vi "stabilizePress_01.vi"() -> ()   [LabVIEW 2011]
uses:
  <vilib>/Platform/TimedLoop/XDataNode/timing_clust.ctl
  <vilib>/Platform/TimedLoop/XDataNode/nitl_modes.ctl
  <vilib>/Platform/TimedLoop/XDataNode/wakeup.ctl
  <vilib>/Platform/TimedLoop/XDataNode/XDataNode.xnode
  <vilib>/Platform/TimedLoop/XDataNode/XDNodeRunTimeDep.lvlib
  <vilib>/Analysis/NI_AALPro.lvlib
panel:
  in  "dtRamp (s)":i64=2
  in  "local when done":bool=TRUE
  out "Best Exponential Fit":dbl[](array[numeric])=[20.391769446914367, 19.671893548435698, 19.339647975340863, 19.18630609922805, 19.115533956951577, 19.082870367269678, 19.067795084021366, 19.060832753073868, 19.057626153023538, 19.056144077997605, 19.055460053338074, 19.055144354249524, 19.05499864910115, 19.054931401551084, 19.054900364672562, 19.05488604016814, 19.054879428954745, 19.05487637564856, 19.054874969405184, 19.054874319446302, 19.05487401946965, 19.054873881020907]
  out "XY Graph":cluster{"Value":dbl[], "Value":dbl[]}[](graph)=[{"Value"=[1.0, 2.0, 3.0, 4.0, 5.0, 6.0, 7.0, 8.001, 9.0, 10.0, 11.0, 12.0, 13.0, 14.0, 15.0, 16.0, 17.0, 18.001, 19.0, 20.0, 21.0, 22.0], "Value"=[20.39, 19.689999999999998, 19.299999999999997, 19.189999999999998, 19.130000000000003, 19.110000000000003, 19.09, 19.08, 19.07, 19.05, 19.04, 19.04, 19.05, 19.05, 19.05, 19.04, 19.05, 19.060000000000002, 19.060000000000002, 19.05, 19.05, 19.05]}, {"Value"=[1.0, 2.0, 3.0, 4.0, 5.0, 6.0, 7.0, 8.001, 9.0, 10.0, 11.0, 12.0, 13.0, 14.0, 15.0, 16.0, 17.0, 18.001, 19.0, 20.0, 21.0, 22.0], "Value"=[20.391769446914367, 19.671893548435698, 19.339647975340863, 19.18630609922805, 19.115533956951577, 19.082870367269678, 19.067795084021366, 19.060832753073868, 19.057626153023538, 19.056144077997605, 19.055460053338074, 19.055144354249524, 19.05499864910115, 19.054931401551084, 19.054900364672562, 19.05488604016814, 19.054879428954745, 19.05487637564856, 19.054874969405184, 19.054874319446302, 19.05487401946965, 19.054873881020907]}]
  out "Pfinal (torr)":dbl=19.054873762353765
  out "tune done":bool=TRUE
  in  "max dP step (torr)":dbl=0.1
  out "dP(torr)":dbl
  out "amplitude":dbl=2.8966495268264136
  out "damping":dbl=-0.7732044604437537
  out "tune Setpoint(torr)":dbl=20.0
  in  "t array":dbl[](array[numeric])=[1.0, 2.0, 3.0, 4.0, 5.0, 6.0, 7.0, 8.001, 9.0, 10.0, 11.0, 12.0, 13.0, 14.0, 15.0, 16.0, 17.0, 18.001, 19.0, 20.0, 21.0, 22.0]
  out "P array":dbl[](array[numeric])=[20.39, 19.689999999999998, 19.299999999999997, 19.189999999999998, 19.130000000000003, 19.110000000000003, 19.09, 19.08, 19.07, 19.05, 19.04, 19.04, 19.05, 19.05, 19.05, 19.04, 19.05, 19.060000000000002, 19.060000000000002, 19.05, 19.05, 19.05]
  out "fit done":bool=TRUE
  in  "tFit(s)":dbl=20.0
  in  "dtFit (s)":i64=1
  out "Set Point (torr)":dbl=20.0 format="%.2f"
  out "Setpoint Index":string="C"
  out "Setpoint Index control":u16(ring)=2 caption="Setpoint" items=["A", "B", "C", "D"]
  out "first":bool
  out "tStart":dbl=22.0
  in  "time done (s)":dbl
  out "Wait to set":bool
  out "IO error":errorcluster
  in  "stop":bool
  out "P (torr)":dbl=19.05 format="%.2f"
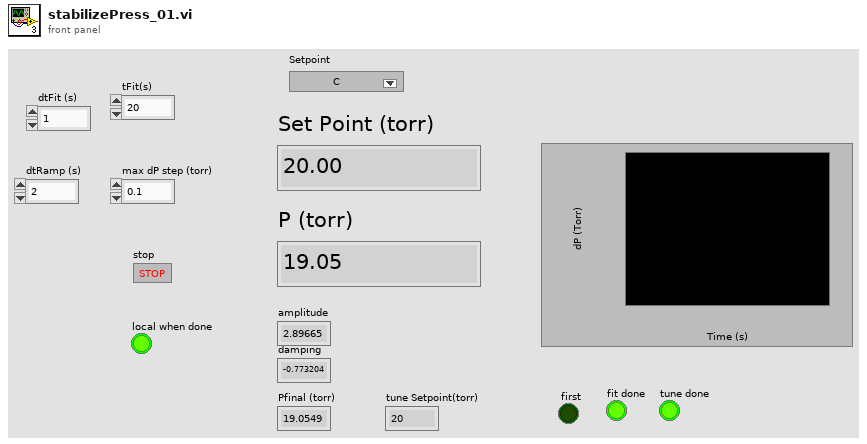
[diagram p1: front panel]
types:
  T1 = typedef "XDNodeRunTimeDep.lvlib/timing_clust.ctl" = cluster{"Expected End [f-1]":u64, "Actual End [f-1]":u64, "Finished Late? [f-1]":bool, "Expected End [i-1]":u64, "Actual End [i-1]":u64, "Finished Late? [i-1]":bool, "Expected Start [i]":u64, "Actual Start [i]":u64, "Expected Start [f]":u64, "Actual Start [f]":u64, "Source Name":string, "Structure Name":string, "Period":i64, "Deadline":i64, "Offset":i64, "Start":i64, "Priority":i32, "Timeout":i32, "Mode":T2, "Wakeup Reason":T3, "Error":errorcluster, "Source Type":string, "Secondary Source Type":string, "Global End Time":u64, "Global Start Time":u64, "Frame Duration":u64, "Iteration Duration":u64, "Assigned CPU":i32, "I/O Scan Engine Mode":u32}
  T2 = typedef "XDNodeRunTimeDep.lvlib/nitl_modes.ctl" = enum32{"No Change", "Process missed periods, maintain original phase", "Discard missed periods, maintain original phase", "Process missed periods, ignore original phase", "Discard missed periods, ignore original phase"}
  T3 = typedef "XDNodeRunTimeDep.lvlib/wakeup.ctl" = enum32{"Normal", "Aborted", "Asynchronous wakeup", "Timing source error", "Timed loop error", "Timeout"}
  T4 = cluster{"amp min":dbl, "amp max":dbl, "damping min":dbl, "damping max":dbl, "offset min":dbl, "offset max":dbl}
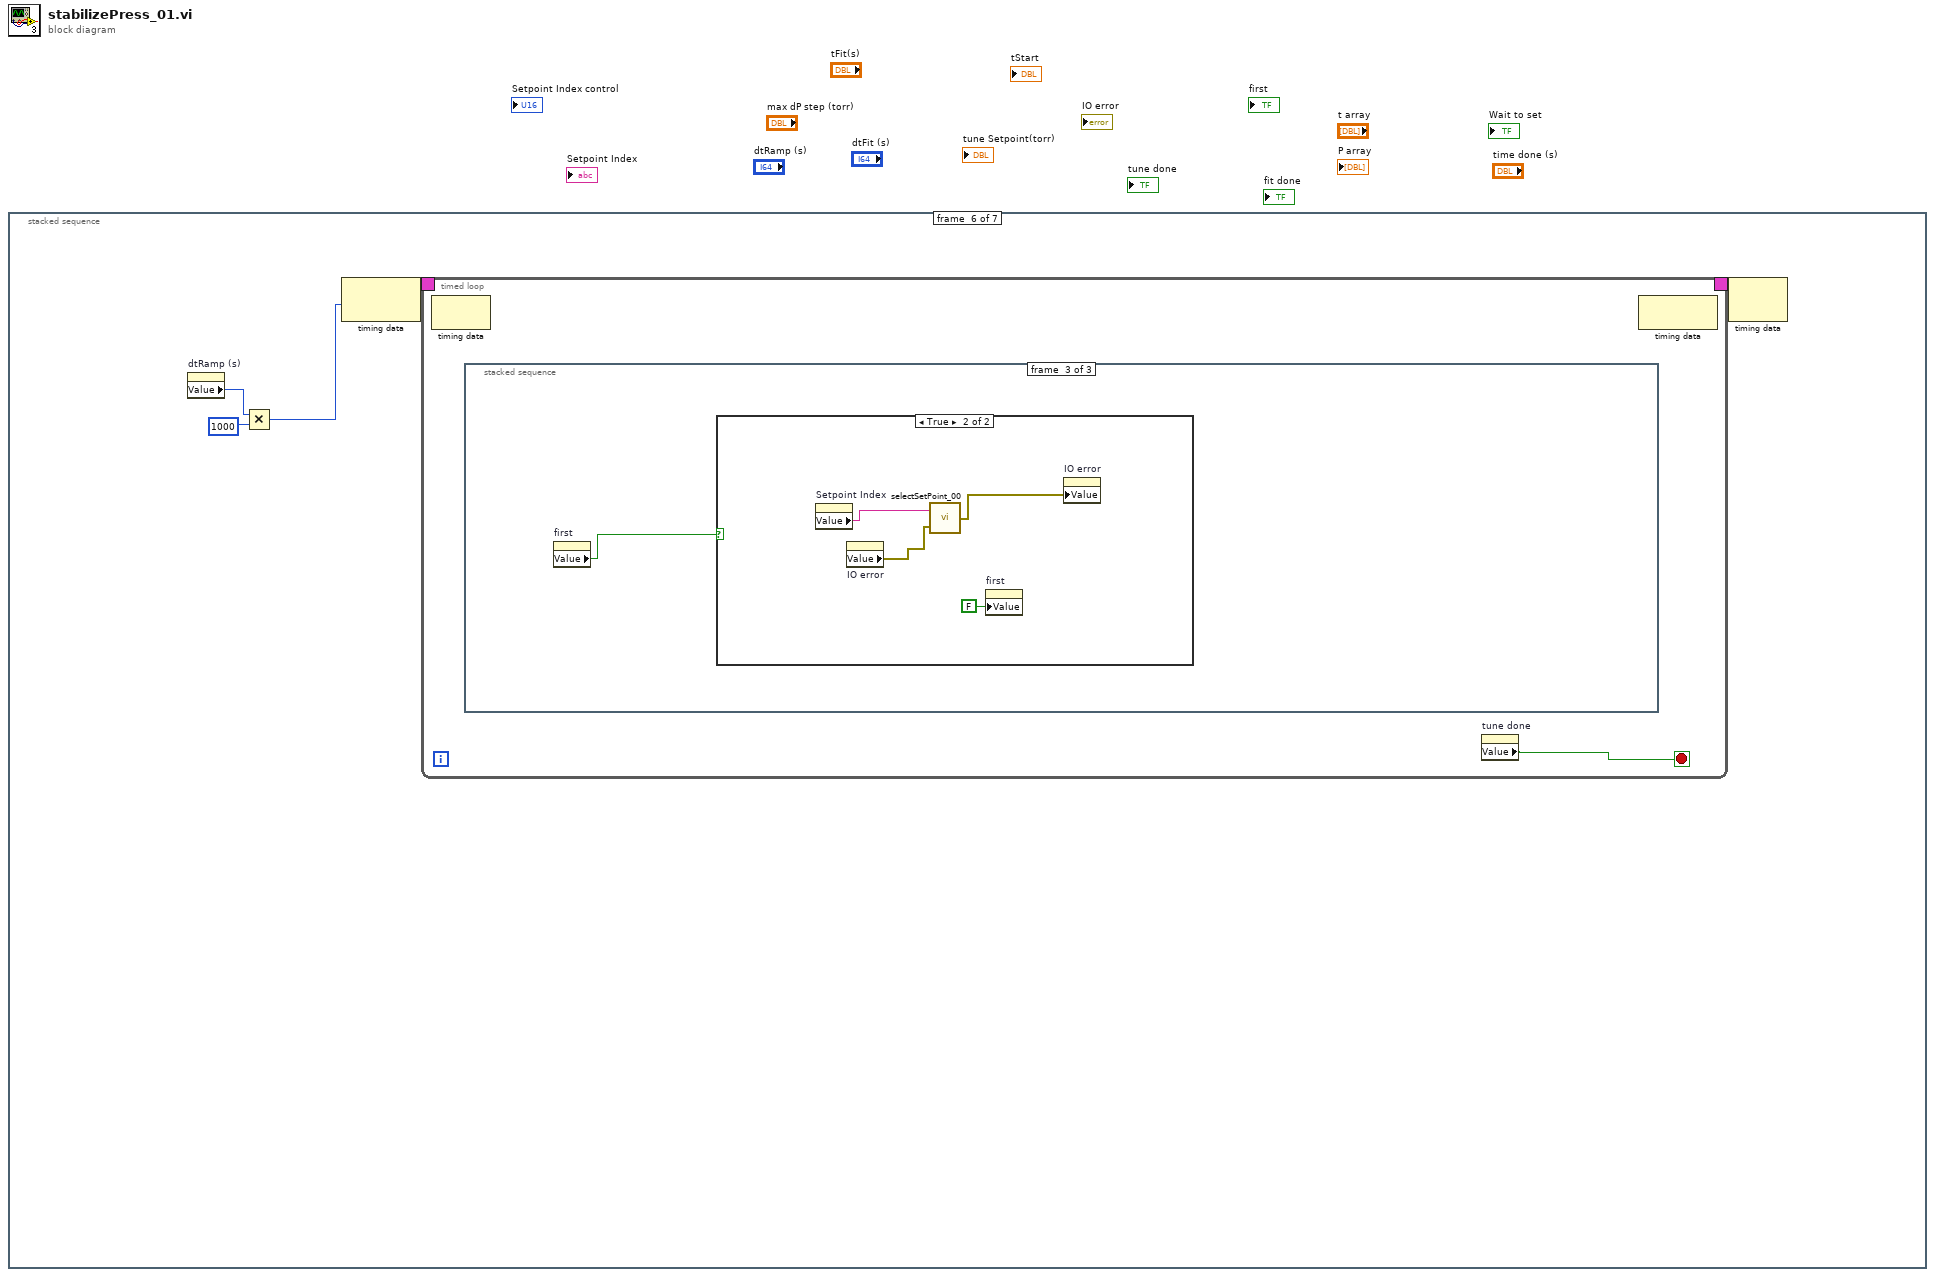
[diagram p0: block diagram]
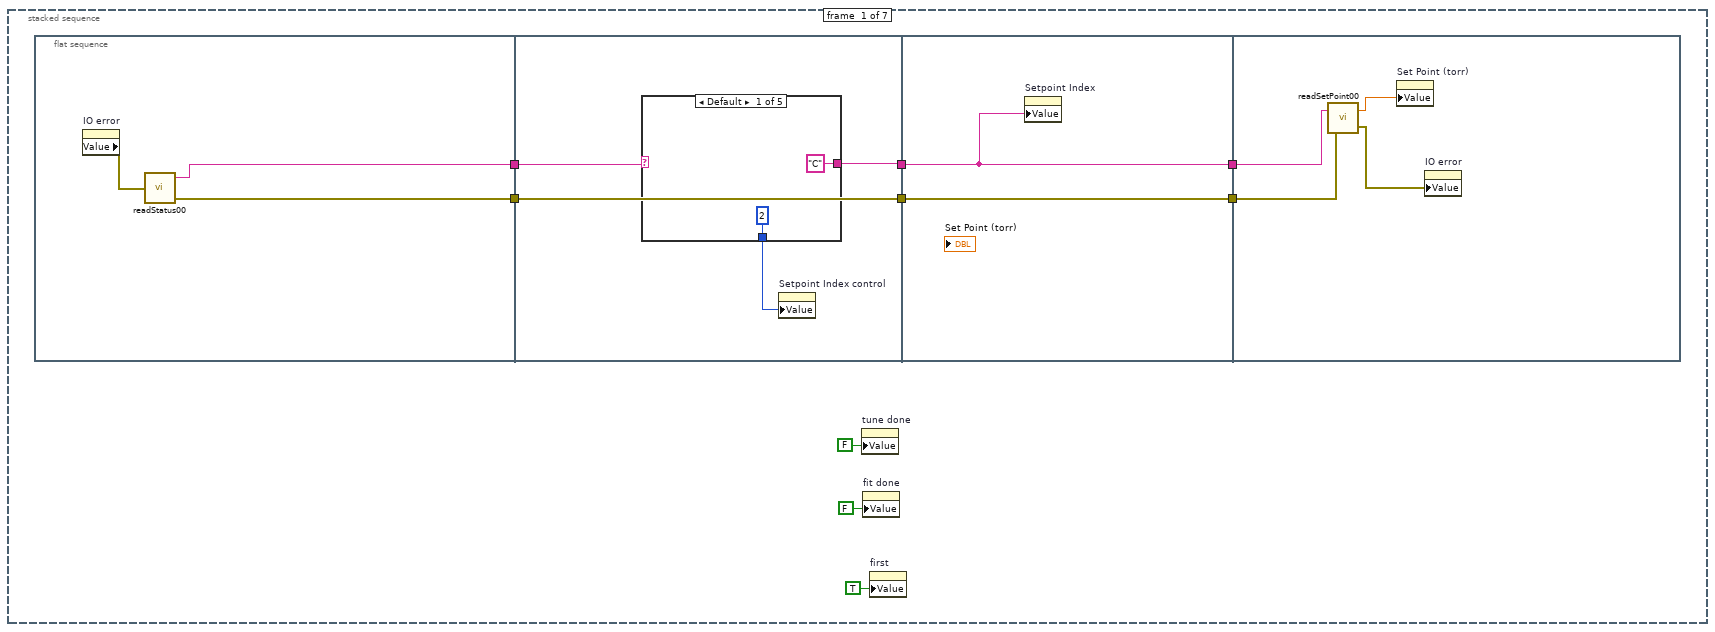
[diagram p2: hidden frame]
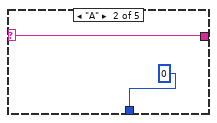
[diagram p3: hidden frame]
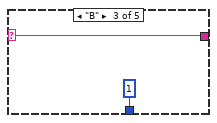
[diagram p4: hidden frame]
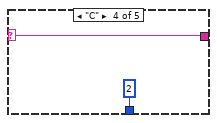
[diagram p5: hidden frame]
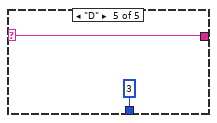
[diagram p6: hidden frame]
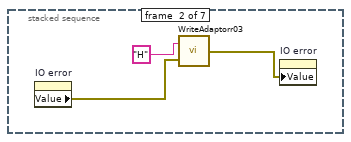
[diagram p7: hidden frame]
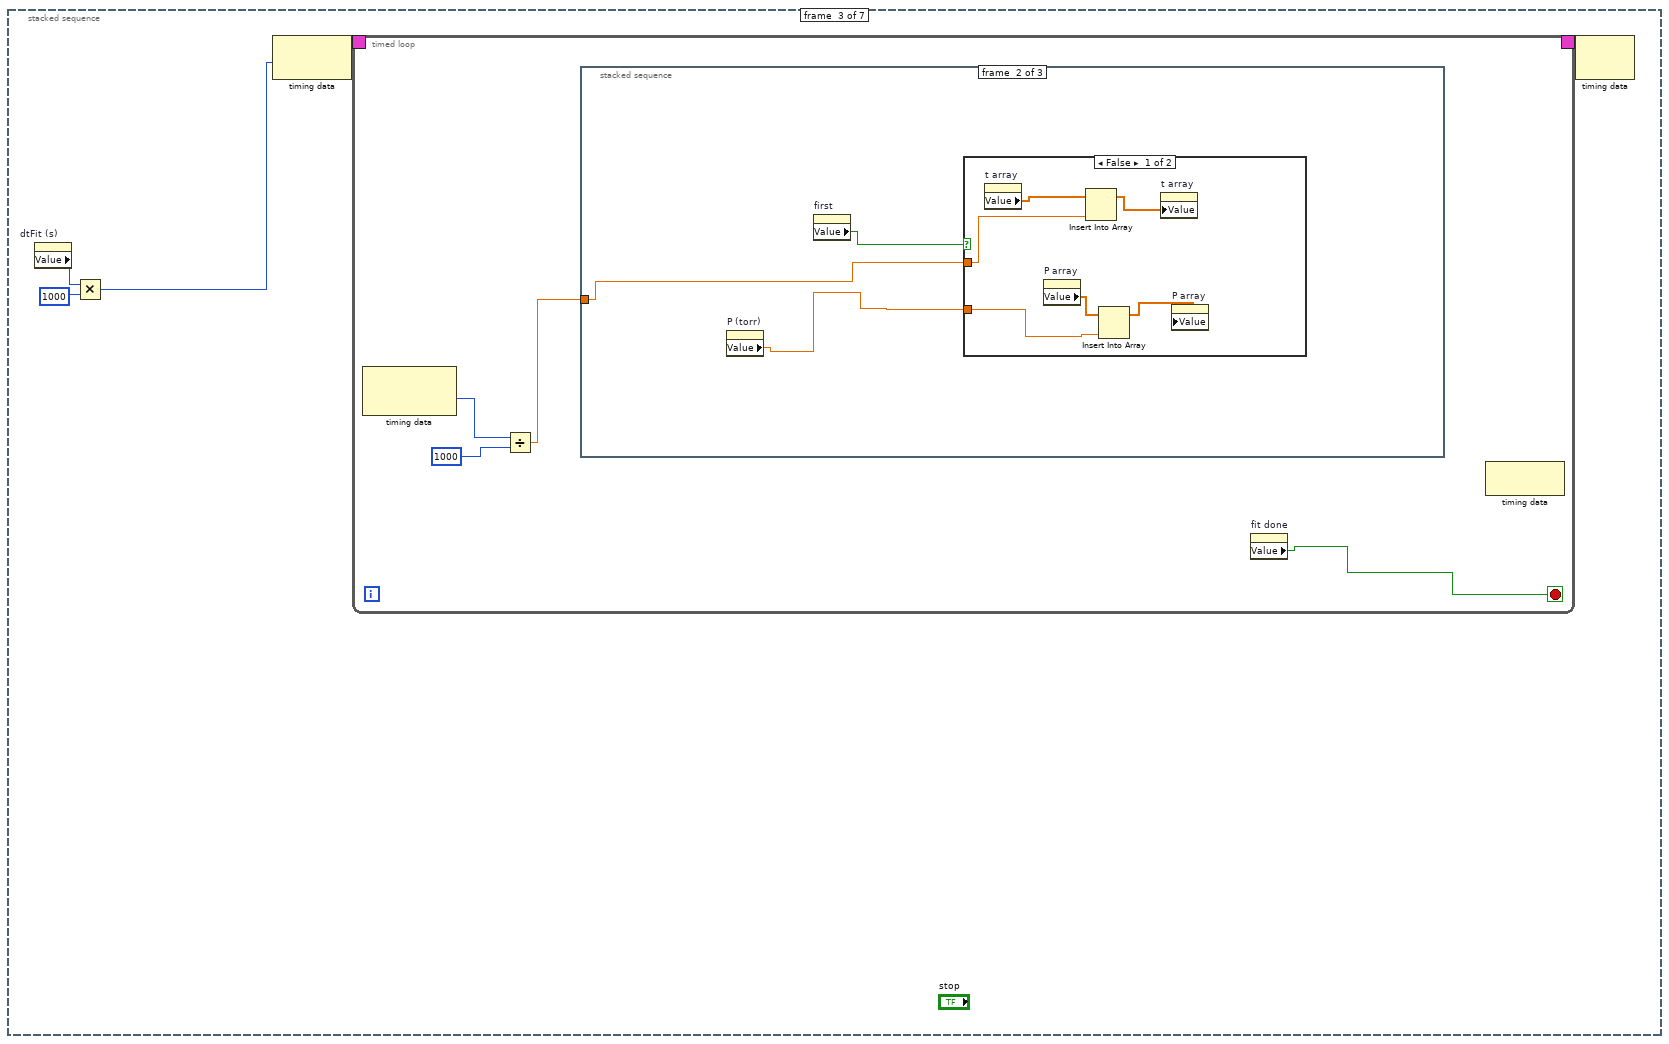
[diagram p8: hidden frame]
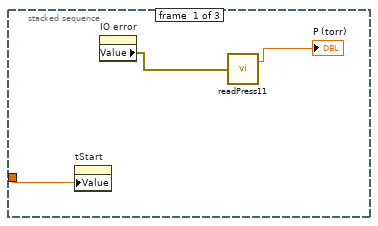
[diagram p9: hidden frame]
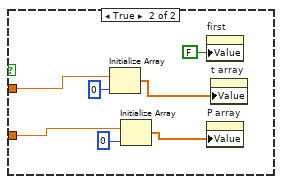
[diagram p10: hidden frame]
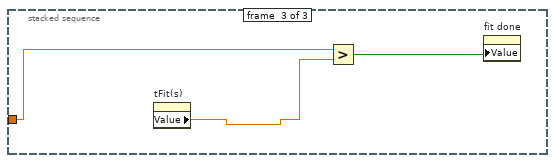
[diagram p11: hidden frame]
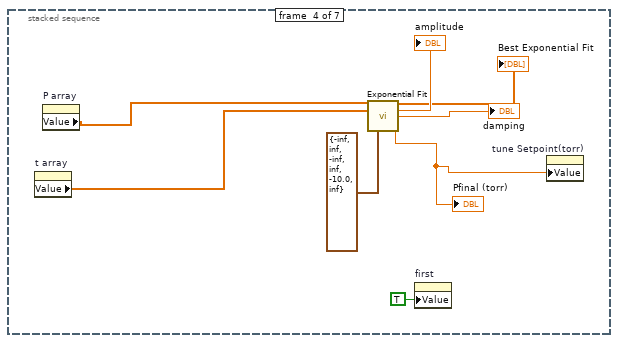
[diagram p12: hidden frame]
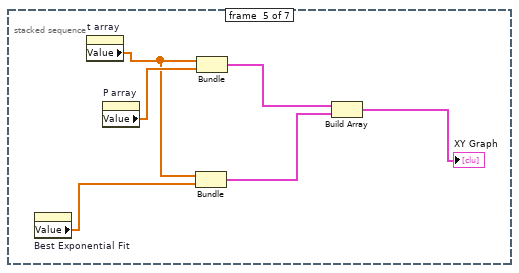
[diagram p13: hidden frame]
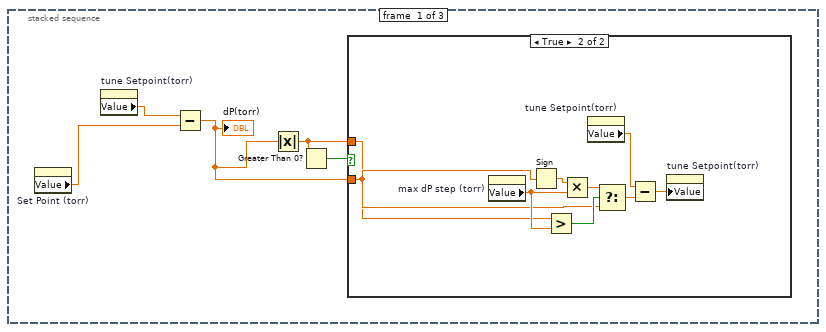
[diagram p14: hidden frame]
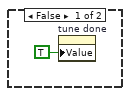
[diagram p15: hidden frame]
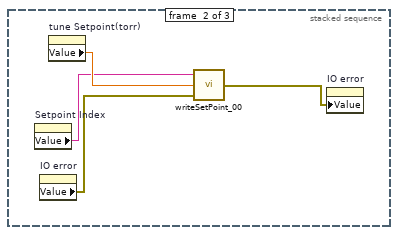
[diagram p16: hidden frame]
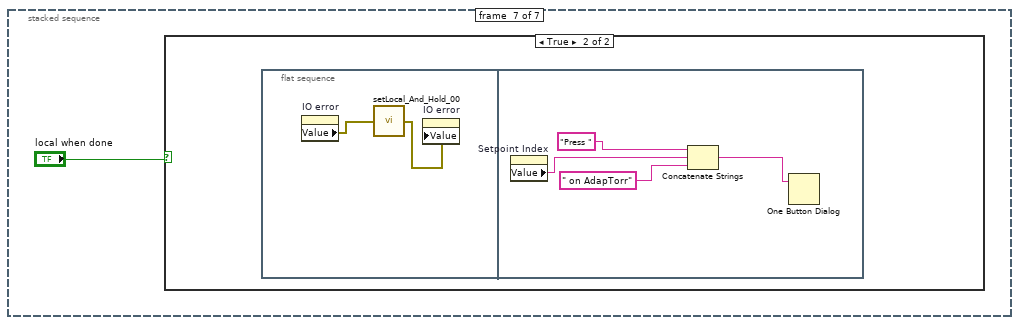
[diagram p18: hidden frame]
diagram:
  n1 = stacked-sequence {
    frame #0 {
      n2 = flat-sequence {
        tunnel: [w11] -> w9
        tunnel: [w10] -> w8
        tunnel: w9 -> [w15]
        tunnel: [w14] -> w7
        tunnel: w8 -> [w16]
        tunnel: [w16] -> w6
        tunnel: w7 -> [w27]
        tunnel: [w27] -> w5
        tunnel: w6 -> [w28]
        tunnel: [w28] -> w4
        tunnel: w5 -> [w32]
        tunnel: w4 -> [w31]
        frame #0 {
          n3 = property on="IO error" class="Clust (strict)"() -> ("Value"=w12:errorcluster)  [unwired: 2 in, 2 out]
          n4 = call "readStatus00.vi"("error in"=w12) -> ("Setpoint"=w11:string, "error out"=w10:errorcluster)  [unwired: 1 out]
        }
        frame #1 {
          n5 = case shown="Default" w15 {
            selector: w15 -> [_ w20 w21 w23 w25]
            tunnel: ["C" w20 w21 w23 w25] -> w14
            tunnel: [u16 2 ("Ring") u16 0 ("Ring") u16 1 ("Ring") u16 2 ("Ring") u16 3 ("Ring")] -> w13
            frame Default {
            }
            frame "A" {
            }
            frame "B" {
            }
            frame "C" {
            }
            frame "D" {
            }
          }
          n6 = property on="Setpoint Index control" class="Ring (strict)"("Value"=w13) -> ()  [unwired: 2 in, 2 out]
        }
        frame #2 {
          n7 = property on="Setpoint Index" class="Str"("Value"=w27) -> ()  [unwired: 2 in, 2 out]
        }
        frame #3 {
          n8 = call "readSetPoint00.vi"("error in"=w31, "Setpoint"=w32) -> ("error out"=w30:errorcluster, "P"=w29:dbl)
          n9 = property on="Set Point (torr)" class="DigNum (strict)"("Value"=w29) -> ()  [unwired: 2 in, 2 out]
          n10 = property on="IO error" class="Clust (strict)"("Value"=w30) -> ()  [unwired: 2 in, 2 out]
        }
      }
      n11 = property on="tune done" class="Bool (strict)"("Value"=FALSE ("tune done")) -> ()  [unwired: 2 in, 2 out]
      n12 = property on="fit done" class="Bool (strict)"("Value"=FALSE ("fit done")) -> ()  [unwired: 2 in, 2 out]
      n13 = property on="first" class="Bool (strict)"("Value"=TRUE ("first")) -> ()  [unwired: 2 in, 2 out]
    }
    frame #1 {
      n14 = property on="IO error" class="Clust (strict)"() -> ("Value"=w34:errorcluster)  [unwired: 2 in, 2 out]
      n15 = call "WriteAdaptorr03.vi"("error in (no error)"=w34, "string to write"="H") -> ("error out"=w33:errorcluster)
      n16 = property on="IO error" class="Clust (strict)"("Value"=w33) -> ()  [unwired: 2 in, 2 out]
    }
    frame #2 {
      n17 = property on="dtFit (s)" class="DigNum (strict)"() -> ("Value"=w37:i64)  [unwired: 2 in, 2 out]
      n18 = Multiply(x=w37, y=u32 1000) -> (x*y=w36:i64)
      n19 = node-c288(w36) -> (w40:T1)
      n20 = timed-loop {
        timing: w40 -> [_]
        timing-out: [_] -> w39
        stop <- w41 stop-if-true
        n21 = node-c288() -> (w44:i64)  [unwired: 1 in, 1 out]
        n22 = Divide(x=w44, y=i64 1000) -> (x/y=w42:dbl)
        n23 = stacked-sequence {
          tunnel: w42 -> [w47 w48 w66]
          frame #0 {
            n24 = property on="tStart" class="DigNum (strict)"("Value"=w47) -> ()  [unwired: 2 in, 2 out]
            n25 = property on="IO error" class="Clust (strict)"() -> ("Value"=w45:errorcluster)  [unwired: 2 in, 2 out]
            n26 = call "readPress11.vi"("error in"=w45) -> ("P"=→"P (torr)":dbl)  [unwired: 1 out]
          }
          frame #1 {
            n27 = property on="P (torr)" class="DigNum (strict)"() -> ("Value"=w49:dbl)  [unwired: 2 in, 2 out]
            n28 = property on="first" class="Bool (strict)"() -> ("Value"=w50:bool)  [unwired: 2 in, 2 out]
            n29 = case shown="False" w50 {
              tunnel: w49 -> [w56 w62]
              tunnel: w48 -> [w53 w60]
              frame False {
                n30 = property on="t array" class="Arr (strict)"() -> ("Value"=w52:dbl[])  [unwired: 2 in, 2 out]
                n31 = property on="P array" class="Arr (strict)"() -> ("Value"=w54:dbl[])  [unwired: 2 in, 2 out]
                n32 = Insert Into Array(array=w52, new element=w53) -> (w51:dbl[])  [unwired: 1 in]
                n33 = Insert Into Array(array=w54, new element=w56) -> (w55:dbl[])  [unwired: 1 in]
                n34 = property on="t array" class="Arr (strict)"("Value"=w51) -> ()  [unwired: 2 in, 2 out]
                n35 = property on="P array" class="Arr (strict)"("Value"=w55) -> ()  [unwired: 2 in, 2 out]
              }
              frame True {
                n36 = Initialize Array(w60, 0 ("dimension size")) -> (w57:dbl[])
                n37 = Initialize Array(w62, 0 ("dimension size")) -> (w58:dbl[])
                n38 = property on="first" class="Bool (strict)"("Value"=FALSE ("first")) -> ()  [unwired: 2 in, 2 out]
                n39 = property on="P array" class="Arr (strict)"("Value"=w58) -> ()  [unwired: 2 in, 2 out]
                n40 = property on="t array" class="Arr (strict)"("Value"=w57) -> ()  [unwired: 2 in, 2 out]
              }
            }
          }
          frame #2 {
            n41 = property on="tFit(s)" class="DigNum (strict)"() -> ("Value"=w64:dbl)  [unwired: 2 in, 2 out]
            n42 = Greater?(x=w66, y=w64) -> (0:w65:bool)
            n43 = property on="fit done" class="Bool (strict)"("Value"=w65) -> ()  [unwired: 2 in, 2 out]
          }
        }
        n44 = property on="fit done" class="Bool (strict)"() -> ("Value"=w41:bool)  [unwired: 2 in, 2 out]
        n45 = node-c288() -> ()  [unwired: 1 in, 1 out]
      }
      n46 = node-c288(w39) -> ()  [unwired: 1 out]
    }
    frame #3 {
      n47 = property on="t array" class="Arr (strict)"() -> ("Value"=w80:dbl[])  [unwired: 2 in, 2 out]
      n48 = property on="P array" class="Arr (strict)"() -> ("Value"=w81:dbl[])  [unwired: 2 in, 2 out]
      n49 = call <vilib>:"Exponential Fit.vi"("Y"=w81, "X"=w80, "parameter bounds"=T4 {"amp min"=-inf, "amp max"=inf, "damping min"=-inf, "damping max"=inf, "offset min"=-10.0, "offset max"=inf}) -> ("Best Exponential Fit"=→"Best Exponential Fit":dbl[], "amplitude"=→"amplitude":dbl, "damping"=→"damping":dbl, "offset"=w77:dbl)  [unwired: 7 in, 2 out]
      "Pfinal (torr)" <- w77
      n50 = property on="first" class="Bool (strict)"("Value"=TRUE ("first")) -> ()  [unwired: 2 in, 2 out]
      n51 = property on="tune Setpoint(torr)" class="DigNum (strict)"("Value"=w77) -> ()  [unwired: 2 in, 2 out]
    }
    frame #4 {
      n52 = property on="Best Exponential Fit" class="Arr (strict)"() -> ("Value"=w85:dbl[])  [unwired: 2 in, 2 out]
      n53 = property on="t array" class="Arr (strict)"() -> ("Value"=w86:dbl[])  [unwired: 2 in, 2 out]
      n54 = property on="P array" class="Arr (strict)"() -> ("Value"=w87:dbl[])  [unwired: 2 in, 2 out]
      n55 = Bundle "Bundle"("Value"=w86, "Value"=w85) -> (w83:cluster{"Value":dbl[], "Value":dbl[]})  [unwired: 1 in]
      n56 = Bundle "Bundle"("Value"=w86, "Value"=w87) -> (w84:cluster{"Value":dbl[], "Value":dbl[]})  [unwired: 1 in]
      n57 = Build Array "Build Array"(w84, w83) -> (→"XY Graph":cluster{"Value":dbl[], "Value":dbl[]}[])
    }
    frame #5 {
      n58 = property on="dtRamp (s)" class="DigNum (strict)"() -> ("Value"=w88:i64)  [unwired: 2 in, 2 out]
      n59 = Multiply(x=w88, y=u32 1000) -> (x*y=w89:i64)
      n60 = node-c288(w89) -> (w92:T1)
      n61 = timed-loop {
        timing: w92 -> [_]
        timing-out: [_] -> w91
        stop <- w93 stop-if-true
        n62 = node-c288() -> ()  [unwired: 1 in, 1 out]
        n63 = stacked-sequence {
          frame #0 {
            n64 = property on="Set Point (torr)" class="DigNum (strict)"() -> ("Value"=w98:dbl)  [unwired: 2 in, 2 out]
            n65 = property on="tune Setpoint(torr)" class="DigNum (strict)"() -> ("Value"=w97:dbl)  [unwired: 2 in, 2 out]
            n66 = Subtract(x=w97, y=w98) -> (x-y=w96:dbl)
            "dP(torr)" <- w96
            n67 = Absolute Value(x=w96) -> (abs(x)=w95:dbl)
            n68 = Greater Than 0?(x=w95) -> (x > 0?=w94:bool)
            n69 = case shown="True" w94 {
              tunnel: w96 -> [_ w104]
              tunnel: w95 -> [_ w100]
              frame False {
                n70 = property on="tune done" class="Bool (strict)"("Value"=TRUE ("tune done")) -> ()  [unwired: 2 in, 2 out]
              }
              frame True {
                n71 = property on="max dP step (torr)" class="DigNum (strict)"() -> ("Value"=w106:dbl)  [unwired: 2 in, 2 out]
                n72 = Sign(1:w104) -> (0:w107:dbl)
                n73 = Greater?(x=w100, y=w106) -> (0:w108:bool)
                n74 = Multiply(x=w107, y=w106) -> (x*y=w105:dbl)
                n75 = property on="tune Setpoint(torr)" class="DigNum (strict)"() -> ("Value"=w103:dbl)  [unwired: 2 in, 2 out]
                n76 = Select(t=w105, s=w108, f=w104) -> (s? t:f=w102:dbl)
                n77 = Subtract(x=w103, y=w102) -> (x-y=w101:dbl)
                n78 = property on="tune Setpoint(torr)" class="DigNum (strict)"("Value"=w101) -> ()  [unwired: 2 in, 2 out]
              }
            }
          }
          frame #1 {
            n79 = property on="Setpoint Index" class="Str"() -> ("Value"=w111:string)  [unwired: 2 in, 2 out]
            n80 = property on="IO error" class="Clust (strict)"() -> ("Value"=w110:errorcluster)  [unwired: 2 in, 2 out]
            n81 = property on="tune Setpoint(torr)" class="DigNum (strict)"() -> ("Value"=w112:dbl)  [unwired: 2 in, 2 out]
            n82 = call "writeSetPoint_00.vi"("error in"=w110, "P (Torr)"=w112, "Setpoint"=w111) -> ("error out"=w109:errorcluster)
            n83 = property on="IO error" class="Clust (strict)"("Value"=w109) -> ()  [unwired: 2 in, 2 out]
          }
          frame #2 {
            n84 = property on="first" class="Bool (strict)"() -> ("Value"=w113:bool)  [unwired: 2 in, 2 out]
            n85 = case shown="True" w113 {
              frame False {
              }
              frame True {
                n86 = property on="Setpoint Index" class="Str"() -> ("Value"=w117:string)  [unwired: 2 in, 2 out]
                n87 = property on="IO error" class="Clust (strict)"() -> ("Value"=w116:errorcluster)  [unwired: 2 in, 2 out]
                n88 = call "selectSetPoint_00.vi"("error in"=w116, "Setpoint"=w117) -> ("error out"=w115:errorcluster)
                n89 = property on="first" class="Bool (strict)"("Value"=FALSE ("first")) -> ()  [unwired: 2 in, 2 out]
                n90 = property on="IO error" class="Clust (strict)"("Value"=w115) -> ()  [unwired: 2 in, 2 out]
              }
            }
          }
        }
        n91 = property on="tune done" class="Bool (strict)"() -> ("Value"=w93:bool)  [unwired: 2 in, 2 out]
        n92 = node-c288() -> ()  [unwired: 1 in, 1 out]
      }
      n93 = node-c288(w91) -> ()  [unwired: 1 out]
    }
    frame #6 {
      n94 = case shown="True" "local when done" {
        frame False {
        }
        frame True {
          n95 = flat-sequence {
            frame #0 {
              n96 = property on="IO error" class="Clust (strict)"() -> ("Value"=w126:errorcluster)  [unwired: 2 in, 2 out]
              n97 = call "setLocal_And_Hold_00.vi"("error in (no error)"=w126) -> ("error out"=w125:errorcluster)
              n98 = property on="IO error" class="Clust (strict)"("Value"=w125) -> ()  [unwired: 2 in, 2 out]
            }
            frame #1 {
              n99 = property on="Setpoint Index" class="Str"() -> ("Value"=w128:string)  [unwired: 2 in, 2 out]
              n100 = Concatenate Strings("Press ", w128, " on AdapTorr") -> (w127:string)
              n101 = One Button Dialog(message=w127) -> ()  [unwired: 1 in, 1 out]
            }
          }
        }
      }
    }
  }
